vi "WILT Read Data Pop Summary.vi"(9 "Inverter File Headers":string[](array[string])=["Date", "Time (24 Hour Format)", "Cycle Time (Minutes)", "L1 Current (Amps)", "L2 Current (Amps)", "TC Temperature (Deg F)", "Voltage (Volts)", "Voltage-208 (Volts)", "208V Switch (Ohms)"], 10 "WILT Summary Cluster Input in":T1, 11 "Log Inverter File":path) -> (3 "WILT Summary Cluster Input out":T1)   [LabVIEW 2016]
uses:
  Type Definitions/WILT Summary Data.ctl
  <vilib>/Utility/file.llb/Read From Spreadsheet File (string).vi
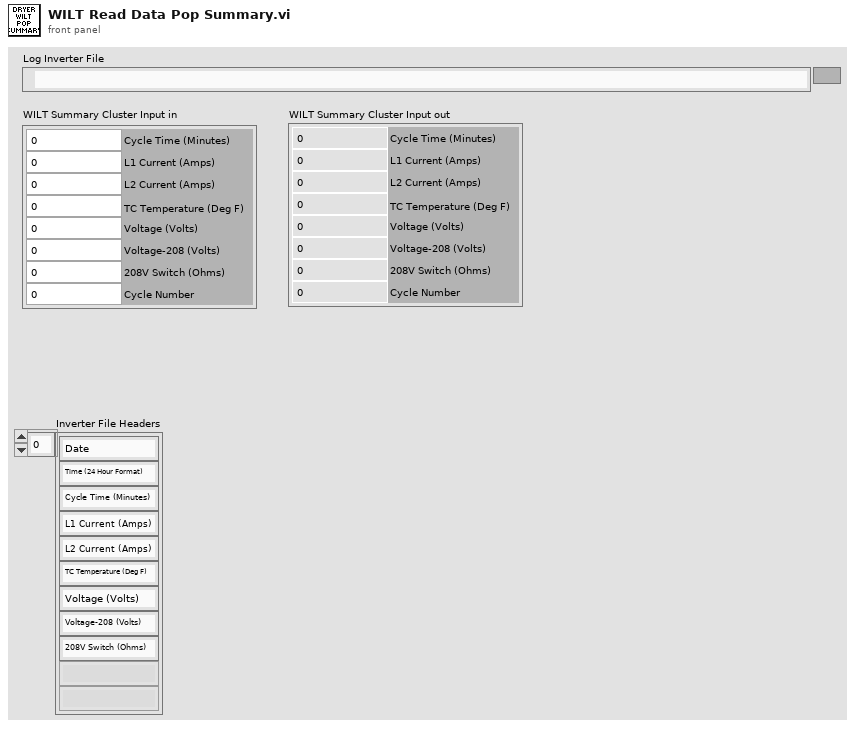
[diagram p1: front panel]
types:
  T1 = typedef "WILT Summary Data.ctl" = cluster{"Cycle Time (Minutes)":dbl, "L1 Current (Amps)":dbl, "L2 Current (Amps)":dbl, "TC Temperature (Deg F)":dbl, "Voltage (Volts)":dbl, "Voltage-208 (Volts)":dbl, "208V Switch (Ohms)":dbl, "Cycle Number":i32}
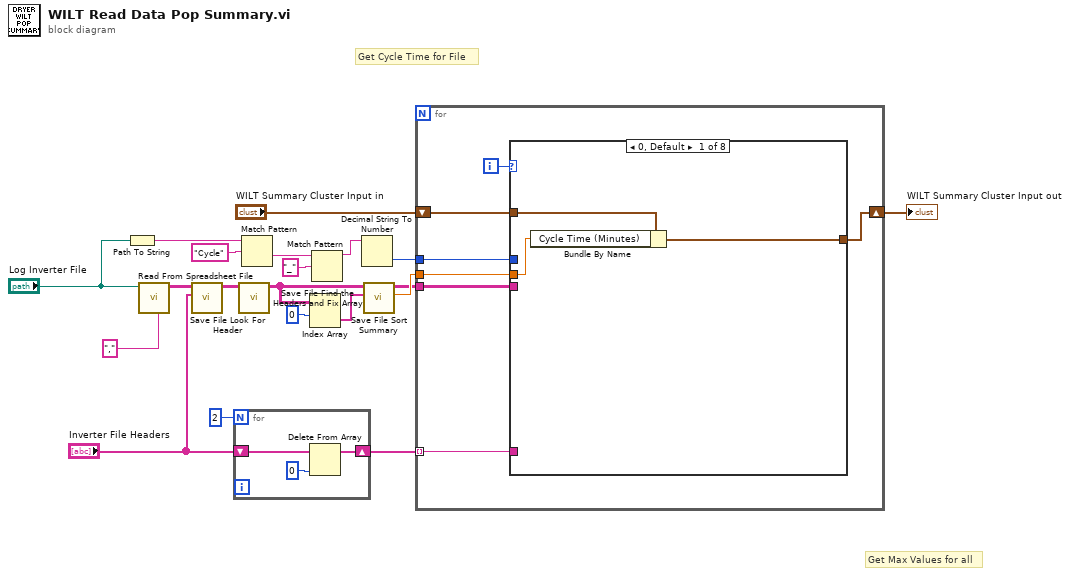
[diagram p0: block diagram]
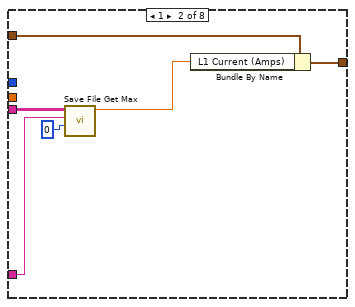
[diagram p2: hidden frame]
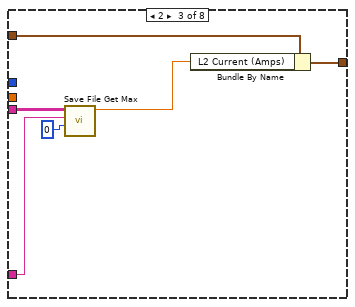
[diagram p3: hidden frame]
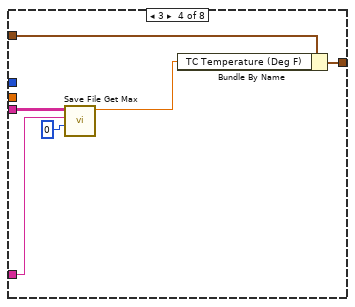
[diagram p4: hidden frame]
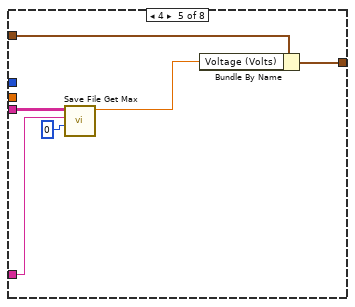
[diagram p5: hidden frame]
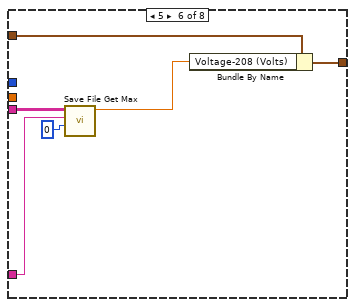
[diagram p6: hidden frame]
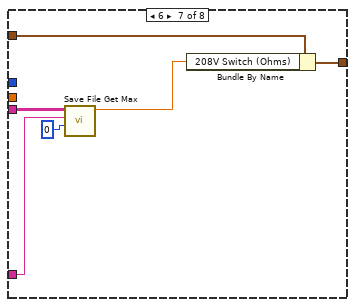
[diagram p7: hidden frame]
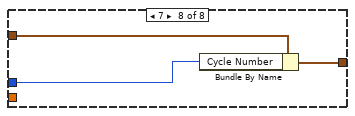
[diagram p8: hidden frame]
diagram:
  # "Get Max Values for all"
  # "Get Cycle Time for File"
  n1 = Path To String(path="Log Inverter File") -> (string=w6:string)
  n2 = call-poly <vilib>:"Read From Spreadsheet File.vi"("delimiter (\\t)"="," ("delimiter (\\t)"), "file path (dialog if empty)"="Log Inverter File") -> ("all rows"=w12:string[][])  [unwired: 5 in, 4 out]
  n3 = call "Save File Look For Header.vi"("Summary Header"="Inverter File Headers", "Full Data IN"=w12) -> ("Data Out"=w13:string[][])  [unwired: 8 in, 1 out]
  n4 = for {
    N: 2 -> [_]
    shift-right: [w22] -> w10
    shift-left: "Inverter File Headers" -> [w23]
    n5 = Delete From Array(array=w23, index=0) -> (array with subset deleted=w22:string[])  [unwired: 1 in, 1 out]
  }
  n6 = call "Save File Find the Headers and Fix Array.vi"("Input"=w13) -> ("Output"=w14:string[][])  [unwired: 9 in, 1 out]
  n7 = Match Pattern(string=w6, regular expression="Cycle") -> (after substring=w4:string)  [unwired: 1 in, 3 out]
  n8 = Index Array(array=w14, index (row)=0) -> (element=w16:string[])  [unwired: 1 in]
  n9 = Match Pattern(string=w4, regular expression="_") -> (before substring=w2:string)  [unwired: 1 in, 3 out]
  n10 = Decimal String To Number(string=w2) -> (number=w1:i32)  [unwired: 2 in, 1 out]
  n11 = call "Save File Sort Summary.vi"("Summary Header"=w16, "Input"=w14) -> ("Cycle Time Minutes"=w18:dbl, "Output"=w17:string[][])  [unwired: 7 in, 1 out]
  n12 = for {
    tunnel: w17 -> [w30]
    tunnel: w10 -> [w29] mode=indexing
    shift-right: [w26] -> w19
    shift-left: "WILT Summary Cluster Input in" -> [w27]
    tunnel: w18 -> [w25]
    tunnel: w1 -> [w24]
    i -> [w28]
    n13 = case shown="0, Default" w28 {
      tunnel: w30 -> [_ w39 w41 w47 w53 w59 w65 _]
      tunnel: w29 -> [_ w37 w40 w46 w52 w58 w64 _]
      tunnel: w27 -> [w33 w36 w44 w50 w56 w61 w67 w72]
      tunnel: [w32 w34 w43 w49 w55 w60 w66 w71] -> w26
      tunnel: w25 -> [w31 _ _ _ _ _ _ _]
      tunnel: w24 -> [_ _ _ _ _ _ _ w70]
      frame 0, Default {
        n14 = Bundle By Name(cluster=w33, "Cycle Time (Minutes)"=w31) -> (w32:T1)
      }
      frame 1 {
        n15 = call "Save File Get Max.vi"("index (row)"=0, "Search Element"=w37, "Full Data"=w39) -> ("Max Value"=w35:dbl)  [unwired: 7 in, 1 out]
        n16 = Bundle By Name(cluster=w36, "L1 Current (Amps)"=w35) -> (w34:T1)
      }
      frame 2 {
        n17 = call "Save File Get Max.vi"("index (row)"=0, "Search Element"=w40, "Full Data"=w41) -> ("Max Value"=w42:dbl)  [unwired: 7 in, 1 out]
        n18 = Bundle By Name(cluster=w44, "L2 Current (Amps)"=w42) -> (w43:T1)
      }
      frame 3 {
        n19 = call "Save File Get Max.vi"("index (row)"=0, "Search Element"=w46, "Full Data"=w47) -> ("Max Value"=w48:dbl)  [unwired: 7 in, 1 out]
        n20 = Bundle By Name(cluster=w50, "TC Temperature (Deg F)"=w48) -> (w49:T1)
      }
      frame 4 {
        n21 = call "Save File Get Max.vi"("index (row)"=0, "Search Element"=w52, "Full Data"=w53) -> ("Max Value"=w54:dbl)  [unwired: 7 in, 1 out]
        n22 = Bundle By Name(cluster=w56, "Voltage (Volts)"=w54) -> (w55:T1)
      }
      frame 5 {
        n23 = call "Save File Get Max.vi"("index (row)"=0, "Search Element"=w58, "Full Data"=w59) -> ("Max Value"=w62:dbl)  [unwired: 7 in, 1 out]
        n24 = Bundle By Name(cluster=w61, "Voltage-208 (Volts)"=w62) -> (w60:T1)
      }
      frame 6 {
        n25 = call "Save File Get Max.vi"("index (row)"=0, "Search Element"=w64, "Full Data"=w65) -> ("Max Value"=w68:dbl)  [unwired: 7 in, 1 out]
        n26 = Bundle By Name(cluster=w67, "208V Switch (Ohms)"=w68) -> (w66:T1)
      }
      frame 7 {
        n27 = Bundle By Name(cluster=w72, "Cycle Number"=w70) -> (w71:T1)
      }
    }
  }
  "WILT Summary Cluster Input out" <- w19
